vi "CreatePlot.vi"(0 "reference in":refnum<class "LcWebView.lvclass">, 5 "Error In":errorcluster, 6 "PlotType":T1) -> (14 "reference out":refnum<class "LcWebView.lvclass">, 19 "Error Out":errorcluster)   [LabVIEW 2019, in "LcWebView.lvclass"]
uses:
  LcWebView.lvclass
  ctrls/PlotType.ctl
  ctrls/PlotRef.ctl
panel:
  out "Loaded":bool
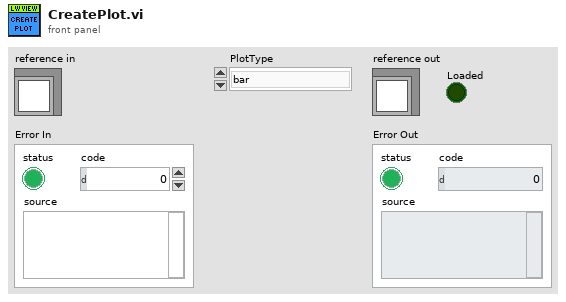
[diagram p1: front panel]
types:
  T1 = typedef "LcWebView.lvclass/PlotType.ctl" = enum16{"bar", "line", "pie"}
  T2 = typedef "LcWebView.lvclass/PlotRef.ctl" = cluster{"PlotType":T1, "PlotTemplate":string}
  T3 = typedef "LcWebView.lvclass/ObjectAttributes.ctl" = cluster{"WebView Container":refnum<k24>, "CoreWebViewRef":refnum<k24>, "Status":i32, "Status Message":string, "User Data Folder":path, "DynamicEvents":T4, "BrowserProcessId":u32, "PlotMap":T5, "PlotType":T1}
  T4 = typedef "LcWebView.lvclass/WebViewDynamicEvents.ctl" = cluster{"Event Registration Ref":refnum<event-registration>, "Source event":refnum<user-event>}
  T5 = typedef "PlotMap.ctl" = map{string, T6}
  T6 = typedef "PlotRef.ctl" = cluster{"PlotType":T1, "PlotTemplate":string}
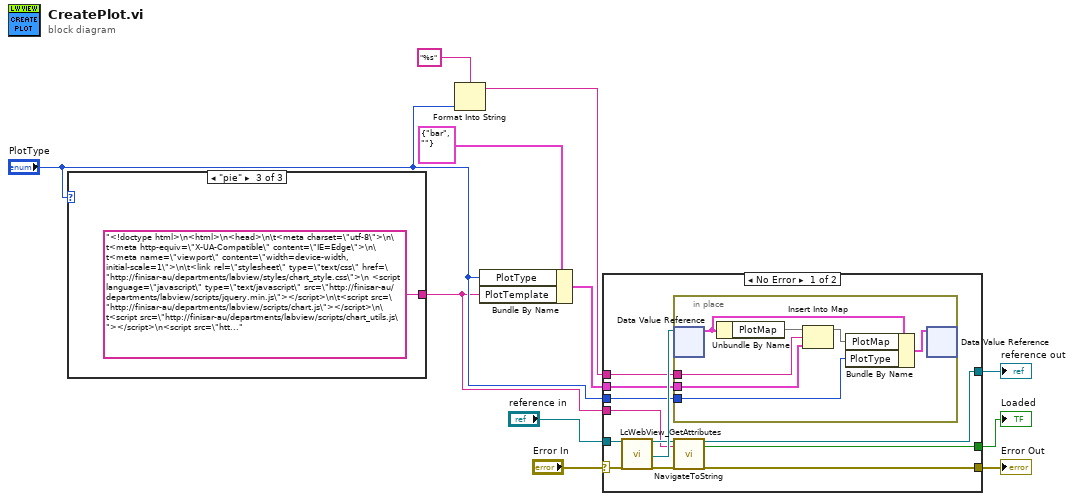
[diagram p0: block diagram]
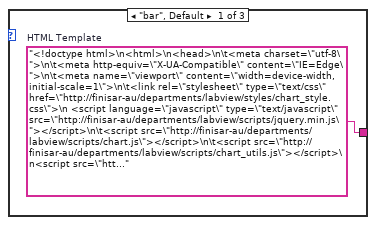
[diagram p2: hidden frame]
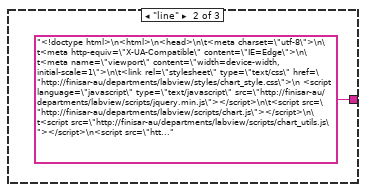
[diagram p3: hidden frame]
diagram:
  n1 = case shown="\"pie\"" "PlotType" {
    tunnel: [w12 "<!doctype html>\n<html>\n<head>\n\t<meta charset=\"utf-8\">\n\t<meta http-equiv=\"X-UA-Compatible\" content=\"IE=Edge\">\n\t<meta name=\"viewport\" content=\"width=device-width, initial-scale=1\">\n\t<link rel=\"stylesheet\" type=\"text/css\" href=\"http://finisar-au/departments/labview/styles/chart_style.css\">\n <script language=\"javascript\" type=\"text/javascript\" src=\"http://finisar-au/departments/labview/scripts/jquery.min.js\"></script>\n\t<script src=\"http://finisar-au/departments/labview/scripts/chart.js\"></script>\n\t<script src=\"http://finisar-au/departments/labview/scripts/chart_utils.js\"></script>\n<script src=\"http://finisar-au/departments/labview/scripts/json2.js\"></script>\n    <script src=\"http://finisar-au/departments/labview/scripts/jquery(v1.11.3).min.js\"></script>\n    <style>\n    \t#container{\n            width:95vm;\n            height:95vh;\n            }\n        #canvas {\n\t\t-moz-user-select: none;\n\t\t-webkit-user-select: none;\n\t\t-ms-user-select: none;  \n\t   }\n\t    </style>\n</head>\n\n<body>\n<div id=\"container\">\n\t\t<canvas id=\"canvas\"></canvas>\n\t</div>\n\t<script type=\"text/javascript\">\n//---colour helper\nvar color = Chart.helpers.color;\nvar plotData ={}  \n\n // summarise config here --------------------------                   \n        var config = {\n\n// **************** PLOT TYPE***************************\n\t\t\ttype: 'line',\n\n\t\t\tdata: plotData,\n//\t\t\t **************** PLOT OPTIONS : THIS PART WILL BE PLOT TYPE DEPENDENT***************************\noptions: \n{\nresponsive: true,\nmaintainAspectRatio: false,\n\t\t\t\tanimation: {\n\t\t\t\t\tanimateScale: true,\n\t\t\t\t\tanimateRotate: true\n\t\t\t\t},\nlegend: {\ndisplay:false,\t\t\t\t\t\t\nposition: 'right'\n\t\t\t\t\t},\ntitle: {\n\t\t\t\t\t\tdisplay:true,\n\t\t\t\t\t\ttext: 'INPUT'\n\t\t\t\t\t},  \n//*************************  ADDITIONAL OPTIONS   ***********************\n\t\t\t\tscales: {\n\t\t\t\t\txAxes: [{\n\t\t\t\t\t\t\tscaleLabel: {\n\t\t\t\t\t\t\tdisplay: true,\n\t\t\t\t\t\t\tlabelString: 'INPUT',\n       stacked:true\n\t\t\t\t\t\t}\n\t\t\t\t\t}],\n\t\t\t\t\tyAxes: [{\n\tticks: {\n\t\t\t\t\t\t\tmin: 0\n\t\t\t\t\t\t\t\t\t\t\t\t\t},\n\t\t\t\t\t\tscaleLabel: {\n\t\t\t\t\t\t\tdisplay: true,\n\t\t\t\t\t\t\tlabelString: 'INPUT',\n       stacked:true\n       \t\t\t\t\t\t}\n\t\t\t\t\t}]\n\t\t\t\t},\ntooltips: {\nenabled: true}\t\n}\n\t\t};\n\nwindow.onload = function() {\n\t  var ctx = document.getElementById('canvas').getContext('2d');\n\t\t\twindow.myChart = new Chart(ctx, config); \n};\nfunction UpdatePlot(data) {        \n            var myData = JSON.parse(data.PlotData);\n            config.data=myData;\n\n            config.options.legend.display= data.GenericPlotOptions.LegendDisplay;\n            config.options.legend.position=data.GenericPlotOptions.LegendPosition;            \n           config.options.title.text=data.GenericPlotOptions.GraphTitle;\n\n//*************************  ADDITIONAL OPTIONS UPDATE ***********************\nconfig.options.scales.yAxes[0].stacked=data.BarPlotOptions.Stacked;\nconfig.options.scales.xAxes[0].stacked=data.BarPlotOptions.Stacked;\nconfig.options.scales.xAxes[0].scaleLabel.labelString=data.BarPlotOptions.xLabel;\nconfig.options.scales.yAxes[0].scaleLabel.labelString=data.BarPlotOptions.yLabel;\nconfig.options.scales.yAxes[0].scaleLabel.display=data.BarPlotOptions.DisplayYLabel;\nconfig.options.scales.xAxes[0].scaleLabel.display=data.BarPlotOptions.DisplayXLabel;\n\n//*************************  UPDATE PLOT ***********************\nwindow.myChart.update();\n\n//*************************  WAIT FOR UPDATE EVENT ***********************\n     }\n\t</script>\n</body>\n</html>" ("HTML Template") "<!doctype html>\n<html>\n<head>\n\t<meta charset=\"utf-8\">\n\t<meta http-equiv=\"X-UA-Compatible\" content=\"IE=Edge\">\n\t<meta name=\"viewport\" content=\"width=device-width, initial-scale=1\">\n\t<link rel=\"stylesheet\" type=\"text/css\" href=\"http://finisar-au/departments/labview/styles/chart_style.css\">\n <script language=\"javascript\" type=\"text/javascript\" src=\"http://finisar-au/departments/labview/scripts/jquery.min.js\"></script>\n\t<script src=\"http://finisar-au/departments/labview/scripts/chart.js\"></script>\n\t<script src=\"http://finisar-au/departments/labview/scripts/chart_utils.js\"></script>\n<script src=\"http://finisar-au/departments/labview/scripts/json2.js\"></script>\n    <script src=\"http://finisar-au/departments/labview/scripts/jquery(v1.11.3).min.js\"></script>\n    <style>\n    \t#container{\n            width:95vm;\n            height:95vh;\n            }\n        #canvas {\n\t\t-moz-user-select: none;\n\t\t-webkit-user-select: none;\n\t\t-ms-user-select: none;  \n\t   }\n\t    </style>\n</head>\n\n<body>\n<div id=\"container\">\n\t\t<canvas id=\"canvas\"></canvas>\n\t</div>\n\t<script type=\"text/javascript\">\n//---colour helper\nvar color = Chart.helpers.color;\nvar plotData ={}  \n\n // summarise config here --------------------------                   \n        var config = {\n\n// **************** PLOT TYPE***************************\n\t\t\ttype: 'pie',\n\n\t\t\tdata: plotData,\n//\t\t\t **************** PLOT OPTIONS : THIS PART WILL BE PLOT TYPE DEPENDENT***************************\noptions: \n{\nresponsive: true,\nmaintainAspectRatio: false,\n\t\t\t\tanimation: {\n\t\t\t\t\tanimateScale: true,\n\t\t\t\t\tanimateRotate: true\n\t\t\t\t},\nlegend: {\ndisplay:false,\t\t\t\t\t\t\nposition: 'right'\n\t\t\t\t\t},\ntitle: {\n\t\t\t\t\t\tdisplay:true,\n\t\t\t\t\t\ttext: 'INPUT'\n\t\t\t\t\t},  \n//*************************  ADDITIONAL OPTIONS   ***********************\ncutoutPercentage:0,\n\ntooltips: {enabled: true,\t\t\t\t\t\ncallbacks: {\n                        title: function(tooltipItems, data) { \n                            var Title= data.datasets[tooltipItems[0].datasetIndex].label\n                            return Title;\n                        },\n\t\t\t// Use the footer callback to display the % of total of the items showing in the tooltip\n                        footer: function(tooltipItems, data) {\n                            console.log(data);\n\t\t\t\t\t\t\tvar ratio = 0;\n                            var sum=0;    \n                            var i=0;\n                            var length = data.datasets[tooltipItems[0].datasetIndex].data.length;\n                            for( i=0;i<length;i++){\n                                sum+= data.datasets[tooltipItems[0].datasetIndex].data[i];\n                            }\n\t\t\t\t\t\t\ttooltipItems.forEach(function(tooltipItem) {\n\t\t\t\t\t\t\t\tratio = 100*data.datasets[tooltipItem.datasetIndex].data[tooltipItem.index]/sum;\n                                ratio=ratio.toFixed(1)\n\t\t\t\t\t\t\t});\n\t\t\t\t\t\t\treturn 'ratio: ' + ratio + '%' ;\n\t\t\t\t\t\t},\n\t\t\t\t\t},\n\t\t\t\t\tfooterFontStyle: 'normal'}\t}\n\t\t};\n\n// run plot function here -------------------------- \nwindow.onload = function() {\n\t  var ctx = document.getElementById('canvas').getContext('2d');\n\t\t\twindow.myChart = new Chart(ctx, config); \n};\nfunction UpdatePlot(data) {        \n            var myData = JSON.parse(data.PlotData);\n            config.data=myData;\n\n            config.options.legend.display= data.GenericPlotOptions.LegendDisplay;\n            config.options.legend.position=data.GenericPlotOptions.LegendPosition;            \n           config.options.title.text=data.GenericPlotOptions.GraphTitle;\n\n//*************************  ADDITIONAL OPTIONS UPDATE ***********************\n config.options.cutoutPercentage=data.PiePlotOptions.cutoutPercentage;\n\n//*************************  UPDATE PLOT ***********************\nwindow.myChart.update();\n\n//*************************  WAIT FOR UPDATE EVENT ***********************\n     }\n\t</script>\n</body>\n</html>" ("HTML Template")] -> w1
    frame "bar", Default {
      w12 = "<!doctype html>\n<html>\n<head>\n\t<meta charset=\"utf-8\">\n\t<meta http-equiv=\"X-UA-Compatible\" content=\"IE=Edge\">\n\t<meta name=\"viewport\" content=\"width=device-width, initial-scale=1\">\n\t<link rel=\"stylesheet\" type=\"text/css\" href=\"http://finisar-au/departments/labview/styles/chart_style.css\">\n <script language=\"javascript\" type=\"text/javascript\" src=\"http://finisar-au/departments/labview/scripts/jquery.min.js\"></script>\n\t<script src=\"http://finisar-au/departments/labview/scripts/chart.js\"></script>\n\t<script src=\"http://finisar-au/departments/labview/scripts/chart_utils.js\"></script>\n<script src=\"http://finisar-au/departments/labview/scripts/json2.js\"></script>\n    <script src=\"http://finisar-au/departments/labview/scripts/jquery(v1.11.3).min.js\"></script>\n    <style>\n    \t#container{\n            width:95vm;\n            height:95vh;\n            }\n        #canvas {\n\t\t-moz-user-select: none;\n\t\t-webkit-user-select: none;\n\t\t-ms-user-select: none;  \n\t   }\n\t    </style>\n</head>\n\n<body>\n<div id=\"container\">\n\t\t<canvas id=\"canvas\"></canvas>\n\t</div>\n\t<script type=\"text/javascript\">\n//---colour helper\nvar color = Chart.helpers.color;\nvar plotData ={}  \n\n // summarise config here --------------------------                   \n        var config = {\n\n// **************** PLOT TYPE***************************\n\t\t\ttype: 'bar',\n\n\t\t\tdata: plotData,\n//\t\t\t **************** PLOT OPTIONS : THIS PART WILL BE PLOT TYPE DEPENDENT***************************\noptions: \n{\nresponsive: true,\nmaintainAspectRatio: false,\n\t\t\t\tanimation: {\n\t\t\t\t\tanimateScale: true,\n\t\t\t\t\tanimateRotate: true\n\t\t\t\t},\nlegend: {\ndisplay:false,\t\t\t\t\t\t\nposition: 'right'\n\t\t\t\t\t},\ntitle: {\n\t\t\t\t\t\tdisplay:true,\n\t\t\t\t\t\ttext: 'INPUT'\n\t\t\t\t\t},  \n//*************************  ADDITIONAL OPTIONS   ***********************\n\t\t\t\tscales: {\n\t\t\t\t\txAxes: [{\n\t\t\t\t\t\t\tscaleLabel: {\n\t\t\t\t\t\t\tdisplay: true,\n\t\t\t\t\t\t\tlabelString: 'INPUT',\n       stacked:true\n\t\t\t\t\t\t}\n\t\t\t\t\t}],\n\t\t\t\t\tyAxes: [{\n\tticks: {\n\t\t\t\t\t\t\tmin: 0\n\t\t\t\t\t\t\t\t\t\t\t\t\t},\n\t\t\t\t\t\tscaleLabel: {\n\t\t\t\t\t\t\tdisplay: true,\n\t\t\t\t\t\t\tlabelString: 'INPUT',\n       stacked:true\n       \t\t\t\t\t\t}\n\t\t\t\t\t}]\n\t\t\t\t},\ntooltips: {\nenabled: true}\t\n}\n\t\t};\n\n// run plot function here -------------------------- \nwindow.onload = function() {\n\t  var ctx = document.getElementById('canvas').getContext('2d');\n\t\t\twindow.myChart = new Chart(ctx, config); \n};\n\nfunction UpdatePlot(data) {        \n    var myData = JSON.parse(data.PlotData);\n    config.data=myData;\n\tconfig.options.legend.display= data.GenericPlotOptions.LegendDisplay;\n\tconfig.options.legend.position=data.GenericPlotOptions.LegendPosition;            \n\tconfig.options.title.text=data.GenericPlotOptions.GraphTitle;\n\n//*************************  ADDITIONAL OPTIONS UPDATE ***********************\n\tconfig.options.scales.yAxes[0].stacked=data.BarPlotOptions.Stacked;\n\tconfig.options.scales.xAxes[0].stacked=data.BarPlotOptions.Stacked;\n\tconfig.options.scales.xAxes[0].scaleLabel.labelString=data.BarPlotOptions.xLabel;\n\tconfig.options.scales.yAxes[0].scaleLabel.labelString=data.BarPlotOptions.yLabel;\n\tconfig.options.scales.yAxes[0].scaleLabel.display=data.BarPlotOptions.DisplayYLabel;\n\tconfig.options.scales.xAxes[0].scaleLabel.display=data.BarPlotOptions.DisplayXLabel;\n\n//*************************  UPDATE PLOT ***********************\n\twindow.myChart.update();\n}\n\t</script>\n</body>\n</html>"  # HTML Template
    }
    frame "line" {
    }
    frame "pie" {
    }
  }
  n2 = Format Into String(format string="%s", "PlotType") -> (resulting string=w5:string)  [unwired: 2 in, 1 out]
  n3 = Bundle By Name(cluster=T2 {"PlotType"=enum."bar", "PlotTemplate"=""} ("PlotRef"), "PlotType"="PlotType", "PlotTemplate"=w1) -> (w4:T2)
  n4 = case shown="No Error" "Error In" {
    selector: "Error In" -> [w26 w35]
    tunnel: [w18 w35] -> w10
    tunnel: [w19 w34] -> w8
    tunnel: "reference in" -> [w25 w34]
    tunnel: w5 -> [w17 _]
    tunnel: w4 -> [w23 _]
    tunnel: "PlotType" -> [w22 _]
    tunnel: [w16 _] -> w3
    tunnel: w1 -> [w15 _]
    frame No Error {
      n5 = call "LcWebView_GetAttributes.vi"("reference in"=w25, "error in (no error)"=w26) -> ("reference out"=w20:refnum<class "LcWebView.lvclass">, "DataRef"=w24:refnum<data-value>, "error out"=w21:errorcluster)  [unwired: 14 in, 1 out]
      n6 = in-place {
        in-place-border: w17 -> [w31]
        in-place-border: w23 -> [w28]
        in-place-border: w22 -> [w27]
        n7 = in-place-dvr #1(w24) -> (w32:T3)  [unwired: 1 out]
        n8 = Unbundle By Name(w32) -> ("PlotMap"=w30:T5)
        n9 = Insert Into Map(map in=w30, key=w31, value=w28) -> (map out=w29:T5)  [unwired: 2 out]
        n10 = Bundle By Name(cluster=w32, "PlotMap"=w29, "PlotType"=w27) -> (w33:T3)
        n11 = in-place-dvr #1(w33) -> ()  [unwired: 2 out]
      }
      n12 = call-dynamic "NavigateToString.vi"("reference in"=w20, "HTML Content"=w15, "Error In"=w21) -> ("reference out"=w19:refnum<class "LcWebView.lvclass">, "Loaded"=w16:bool, "Error Out"=w18:errorcluster)  [unwired: 14 in]
    }
    frame Error {
    }
  }
  "Error Out" <- w10
  "reference out" <- w8
  "Loaded" <- w3
